vi "WaveGraph_UnInit.vi"(2 "Container State":T1 caption="容器状态", 3 "Display State":T2 caption="显示状态") -> ()   [LabVIEW 2012, in "WaveGraphX.xctl"]
uses:
  WaveGraphX.xctl
  WaveGraph_State.ctl
  <vilib>/_xctls/Container State.ctl
  <vilib>/_xctls/XControlSupport.lvlib
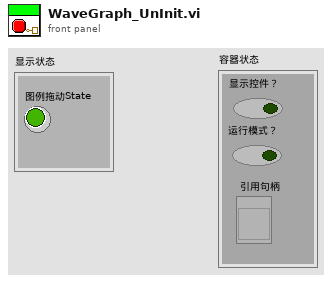
[diagram p1: front panel]
types:
  T1 = typedef "XControlSupport.lvlib/Container State.ctl" = cluster{"Indicator?":bool, "Run Mode?":bool, " Refnum":refnum<vi>}
  T2 = typedef "WaveGraphX.xctl/WaveGraph_State.ctl" = cluster{"图例拖动State":bool}
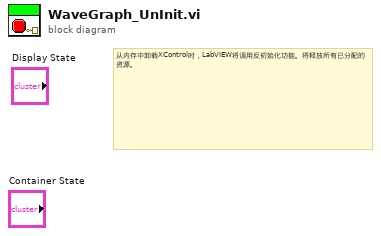
[diagram p0: block diagram]
diagram:
  # "从内存中卸载XControl时，LabVIEW将调用反初始化功能。将释放所有已分配的资源。"
